vi "Agilent PWM Read Blank Screen.vi"(7 "Agilent PWM":T1, 8 "error in (no error)":errorcluster, 11 "VISA Resource Name":refnum<visa-resource-name>) -> (0 "error out":errorcluster, 2 "Blank Screen":bool, 3 "dup VISA Resource Name":refnum<visa-resource-name>)   [LabVIEW 2011]
doc: "This VI for the HP 8753 is used to read the sweep type.\n\n0 LINEAR FREQ\n1 LOG FREQ\n2 LIST FREQ\n3 CW TIME\n4 POWER SWEEP"
uses:
  TypeDefs/Agilent PWM Instrument Info.ctl
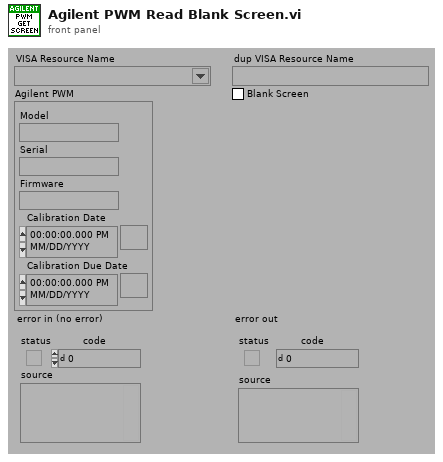
[diagram p1: front panel]
types:
  T1 = typedef "Agilent PWM Instrument Info.ctl" = cluster{"Model":string, "Serial":string, "Firmware":string, "Calibration Date":timestamp, "Calibration Due Date":timestamp}
  T2 = typedef "Agilent PWM Model.ctl" = enum16{"Not Supported", "E4418X", "E4419X", "U2000X"}
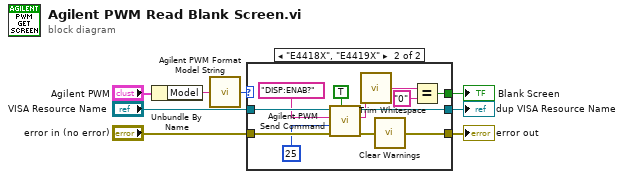
[diagram p0: block diagram]
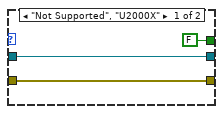
[diagram p2: hidden frame]
diagram:
  n1 = Unbundle By Name("Agilent PWM") -> ("Model"=w2:string)
  n2 = call "Agilent PWM Format Model String.vi"("Model"=w2) -> ("Model"=w1:T2)
  n3 = case shown="\"E4418X\", \"E4419X\"" w1 {
    tunnel: "error in (no error)" -> [w10 w23]
    tunnel: "VISA Resource Name" -> [w11 w22]
    tunnel: [w10 w20] -> w6
    tunnel: [w11 w18] -> w5
    tunnel: [FALSE w12] -> w4
    frame "Not Supported", "U2000X" {
    }
    frame "E4418X", "E4419X" {
      n4 = call "Agilent PWM Send Command.vi"("Read? (F)"=TRUE, "error in (no error)"=w23, "Byte Count"=u32 25 ("byte count"), "Command"="DISP:ENAB?" ("write buffer"), "VISA Resource Name"=w22) -> ("error out"=w19:errorcluster, "Data Read"=w13:string, "dup VISA Resource Name"=w18:refnum<visa-resource-name>)  [unwired: 4 out]
      n5 = call <vilib>:"Trim Whitespace.vi"("string"=w13) -> ("trimmed string"=w14:string)  [unwired: 1 in]
      n6 = call "Clear Warnings.vi"("error in (no error)"=w19) -> ("error out"=w20:errorcluster)
      n7 = Equal?(x=w14, y="0") -> (x = y?=w12:bool)
    }
  }
  "dup VISA Resource Name" <- w5
  "error out" <- w6
  "Blank Screen" <- w4
